vi "Remove Warning.vi"(3 "error in (no error)":errorcluster, 5 "VISA resource name":refnum<visa-resource-name>) -> (0 "error out":errorcluster, 2 "VISA resource name out":refnum<visa-resource-name>)   [LabVIEW 2012, in "MicroStrain 3DM-GXx.lvlib"]
doc: "Removes the following warning: 'The number of bytes transferred is equal to the requested\ninput count'."
uses:
  <instrlib>/MicroStrain 3DM-GXx/MicroStrain 3DM-GXx.lvlib
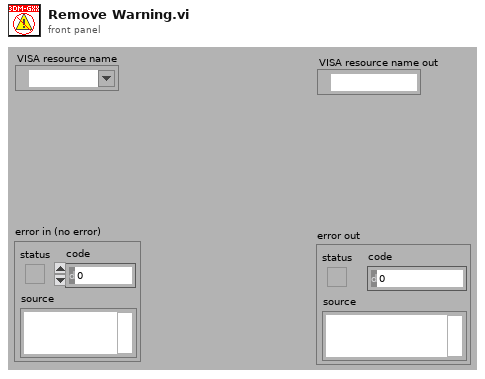
[diagram p1: front panel]
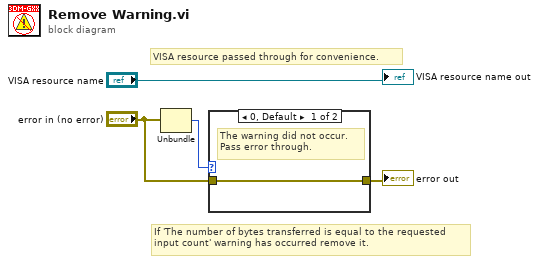
[diagram p0: block diagram]
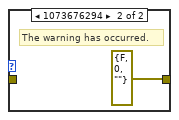
[diagram p2: hidden frame]
diagram:
  # "VISA resource passed through for convenience."
  # "If 'The number of bytes transferred is equal to the requested\ninput count' warning has occurred remove it."
  n1 = Unbundle("error in (no error)") -> ("code"=w4:i32)  [unwired: 2 out]
  n2 = case shown="0, Default" w4 {
    tunnel: "error in (no error)" -> [w5 _]
    tunnel: [w5 errorcluster {"status"=FALSE, "code"=0, "source"=""} ("error in (no error)")] -> w2
    frame 0, Default {
      # "The warning did not occur.\nPass error through."
    }
    frame 1073676294 {
      # "The warning has occurred."
    }
  }
  "error out" <- w2
  "VISA resource name out" <- "VISA resource name"
